vi "Do.vi"(8 "error in (no error)":errorcluster, 10 "Actor in":refnum<class "Actor.lvclass">, 11 "Card_detection Msg":refnum<class "Card_detection Msg.lvclass">) -> (0 "error out":errorcluster, 2 "Actor out":refnum<class "Actor.lvclass">)   [LabVIEW 2025, in "User_Console-ATM.lvlib" / "Card_detection Msg.lvclass"]
doc: "This VI delivers the message to the actor by calling the appropriate method(s) on the actor."
uses:
  Card_detection Msg.lvclass
  Card_detection Msg.lvclass/Card_detection Msg.ctl
  User_Console_States/User_Console_States.lvclass
  C:/Program Files (x86)/National Instruments/LabVIEW 2025/vi.lib/ni/Actors/State Actor/State Actor/State Actor.lvclass
  C:/Program Files (x86)/National Instruments/LabVIEW 2025/vi.lib/ActorFramework/Actor/Actor.lvclass
  C:/Users/halstead_rideriver/Documents/Labview_Practice/ATM_Machine_Actor Framework/ATM_ACTORFW/User_Console-ATM/User_Console_States/User_Console_States.lvclass
  c3dfc7b2-2b44-4ab1-93de-fa5051308527.vi
  <vilib>/ActorFramework/Actor/Actor.lvclass
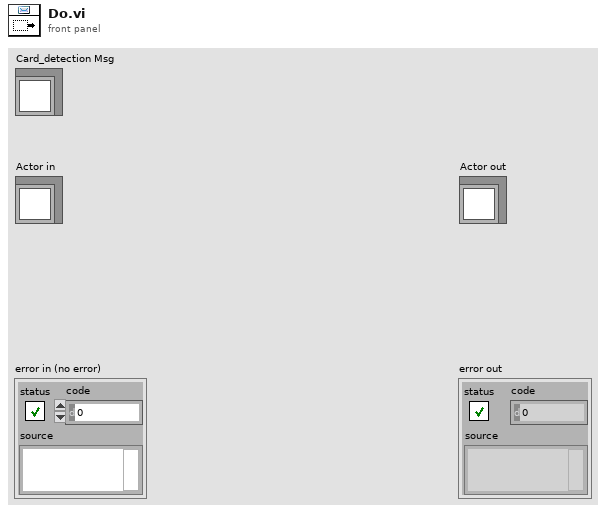
[diagram p1: front panel]
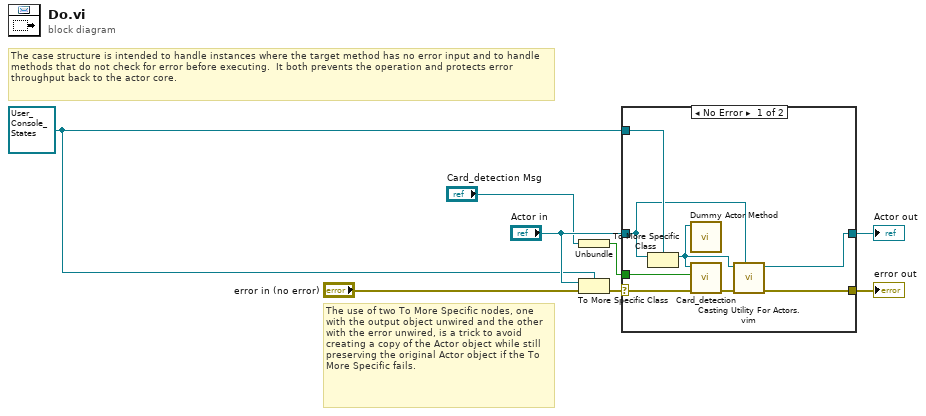
[diagram p0: block diagram]
diagram:
  w3 = refnum<class "User_Console_States.lvclass"> refnum ("Actor in")
  # "The use of two To More Specific nodes, one with the output object unwired and the other with the error unwired, is a trick to avoid creating a copy of the Actor object while still preserving the original Actor object if the To More Specific fails."
  # "The case structure is intended to handle instances where the target method has no error input and to handle methods that do not check for error before executing.  It both prevents the operation and protects error throughput back to the actor core."
  n1 = Unbundle("Card_detection Msg") -> (w1:bool)
  n2 = To More Specific Class(target class=w3, reference="Actor in", error in="error in (no error)") -> (error out=w2:errorcluster)  [unwired: 1 out]
  n3 = case shown="No Error" w2 {
    selector: w2 -> [w16 w18]
    tunnel: [w11 w18] -> w8
    tunnel: [w12 w17] -> w7
    tunnel: "Actor in" -> [w13 w17]
    tunnel: w3 -> [w14 _]
    tunnel: w1 -> [w9 _]
    frame No Error {
      n4 = To More Specific Class(target class=w14, reference=w13) -> (specific class reference=w15:refnum<class "User_Console_States.lvclass">)  [unwired: 1 in, 1 out]
      n5 = call <resource>:"Dummy Actor Method.vi"("Actor in"=w15) -> ()  [unwired: 9 in, 2 out]
      n6 = call-dynamic "Card_detection.vi"("error in (no error)"=w16, "Card"=w9, "User_Console_States in"=w15) -> ("error out"=w10:errorcluster)  [unwired: 7 in, 1 out]
      n7 = call "Casting Utility For Actors.vim"("type"=w13, "error in (no error)"=w10, "Actor in"=w15) -> ("error out"=w11:errorcluster, "Actor out"=w12:refnum<class "Actor.lvclass">)  [unwired: 7 in]
    }
    frame Error {
      # "If type check fails, pass the original object out again."
    }
  }
  "error out" <- w8
  "Actor out" <- w7
